vi "Create Terminal.vi"(7 "Direction":bool, 8 "error in (no error)":errorcluster, 9 "Symbol":refnum<class "Shape.lvclass">, 10 "Text Shape":refnum<class "Text.lvclass">, 11 "Terminal in":refnum<class "Terminal.lvclass">) -> (0 "error out":errorcluster, 3 "Terminal out":refnum<class "Terminal.lvclass">)   [LabVIEW 2015, in "Terminal.lvclass"]
uses:
  Terminal.lvclass
  <vilib>/LIEF/Forms/Text/Text.lvclass
  <vilib>/LIEF/Forms/Shape/Shape.lvclass
  Terminal.lvclass/Terminal.ctl
  <vilib>/LIEF/Forms/Layered Shape/Layered Shape.lvclass/Layered Shape.ctl
  <vilib>/LIEF/Forms/Layered Shape/Write Overlays.vi
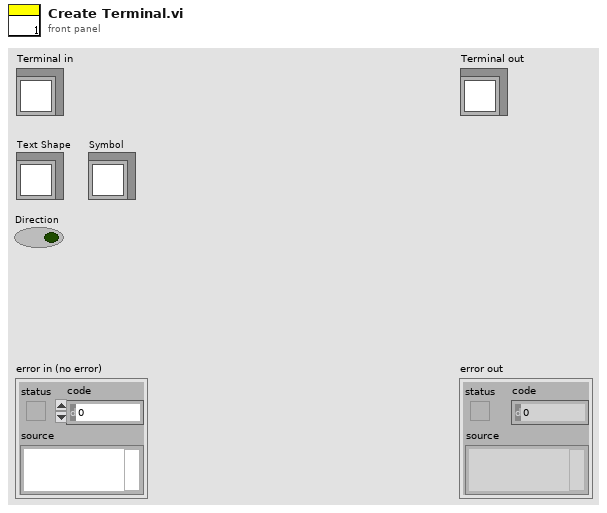
[diagram p1: front panel]
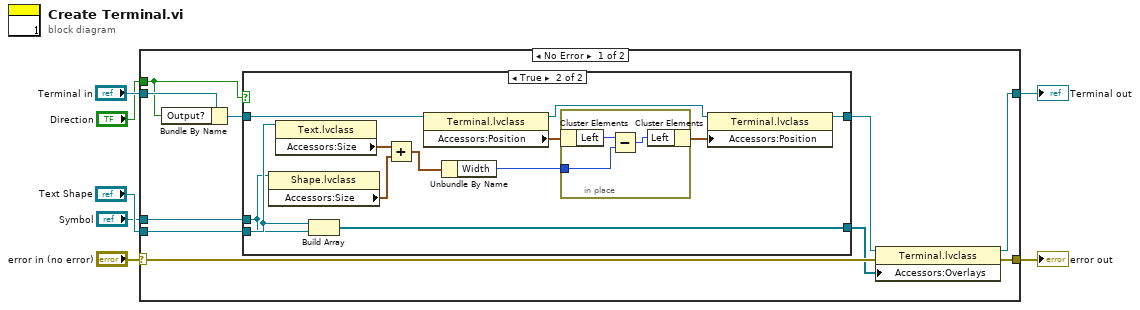
[diagram p0: block diagram]
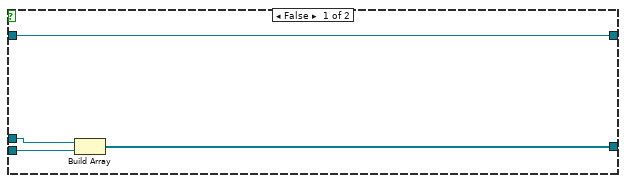
[diagram p2: hidden frame]
diagram:
  n1 = case shown="No Error" "error in (no error)" {
    selector: "error in (no error)" -> [w16 w38]
    tunnel: [w15 w38] -> w6
    tunnel: [w14 w37] -> w4
    tunnel: "Terminal in" -> [w17 w37]
    tunnel: "Text Shape" -> [w12 _]
    tunnel: "Direction" -> [w13 _]
    tunnel: "Symbol" -> [w11 _]
    frame No Error {
      n2 = Bundle By Name(cluster=w17, "Output?"=w13) -> (w9:refnum<class "Terminal.lvclass">)
      n3 = case shown="True" w13 {
        tunnel: w12 -> [w21 w32]
        tunnel: w11 -> [w20 w31]
        tunnel: [w19 w33] -> w10
        tunnel: w9 -> [w18 w30]
        tunnel: [w18 w26] -> w8
        frame False {
          n4 = Build Array(w20, w21) -> (w19:refnum<class "Shape.lvclass">[])
        }
        frame True {
          n5 = property class="Shape.lvclass"(reference=w31) -> ("Accessors:Size"=w29:cluster{"Width":i32, "Height":i32})  [unwired: 1 in, 2 out]
          n6 = property class="Text.lvclass"(reference=w32) -> ("Accessors:Size"=w28:cluster{"Width":i32, "Height":i32})  [unwired: 1 in, 2 out]
          n7 = Build Array(w32, w31) -> (w33:refnum<class "Shape.lvclass">[])
          n8 = Add(x=w28, y=w29) -> (x+y=w24:cluster{"Width":i32, "Height":i32})
          n9 = property class="Terminal.lvclass"(reference=w30) -> (reference out=w27:refnum<class "Terminal.lvclass">, "Accessors:Position"=w25:cluster{"Left":i32, "Top":i32})  [unwired: 1 in, 1 out]
          n10 = Unbundle By Name(w24) -> ("Width"=w23:i32)
          n11 = in-place {
            in-place-border: w23 -> [w35]
            n12 = in-place-cluster #1(w25) -> ("Left"=w36:i32)
            n13 = Subtract(x=w36, y=w35) -> (x-y=w34:i32)
            n14 = in-place-cluster #1("Left"=w34) -> (w22:cluster{"Left":i32, "Top":i32})
          }
          n15 = property class="Terminal.lvclass"(reference=w27, "Accessors:Position"=w22) -> (reference out=w26:refnum<class "Terminal.lvclass">)  [unwired: 1 in, 1 out]
        }
      }
      n16 = property class="Terminal.lvclass"(reference=w8, error in=w16, "Accessors:Overlays"=w10) -> (reference out=w14:refnum<class "Terminal.lvclass">, error out=w15:errorcluster)
    }
    frame Error {
    }
  }
  "error out" <- w6
  "Terminal out" <- w4
